vi "CSM with allowed message list.vi"(7 "Name (\"\" to Use Uuid)":string="Event CSM Tiny") -> ()   [LabVIEW 2017]
doc: "------------- lvcsm -------------\n[CSMStates]\nItem 0 = \"Event Structure\"\nItem 1 = \"Idle\"\nItem 2 = \"CSM Documentation\"\nItem 3 = \"VI Reference\"\nItem 4 = \"Error Handler\"\nItem 5 = \"Critical Error\"\nItem 6 = \"Target Busy Error\"\nItem 7 = \"Target Error\"\nItem 8 = \"Target Timeout Error\"\nItem 9 = \"Async Response\"\nItem 10 = \"Response\"\nItem 11 = \"Async Message Posted\"\nItem 12 = \"Initialize Core Data\"\nItem 13 = \"Exit\"\nItem 14 = \"Data: Initialize\"\nItem 15 = \"Data: Cleanup\"\nItem 16 = \"Events: Register\"\nItem 17 = \"Events: Unregister\"\nItem 18 = \"UI: Initialize\"\nItem 19 = \"UI: Cursor Set\"\nItem 20 = \"UI: Front Panel State\"\nItem 21 = \"Macro: Initialize\"\nItem 22 = \"Macro: Exit\"\nItem 23 = \"API: API1\"\nItem 24 = \"API: API2\"\nItem 25 = \"DoSth: DoA\"\nItem 26 = \"DoSth: DoB\"\n\n[CSMStatus]\nItem 0 = \"Error Occurred@Error Handler\""
uses:
  user.lib/_NEVSTOP/Communicable State Machine(CSM)/AdvanceAPI/CSM - Revert Arguments-Safe String.vi
  user.lib/_NEVSTOP/Communicable State Machine(CSM)/AdvanceAPI/CSM - Break Down Multiple States String.vi
  user.lib/_NEVSTOP/Communicable State Machine(CSM)/AdvanceAPI/CSM - Compact Multiple States.vi
  user.lib/_NEVSTOP/Communicable State Machine(CSM)/AdvanceAPI/CSM - Make String Arguments Safe.vi
  user.lib/_NEVSTOP/Communicable State Machine(CSM)/AdvanceAPI/CSM - Keywords.vi
  user.lib/_NEVSTOP/Communicable State Machine(CSM)/_Shared/Trim Single-line Text.vi
  user.lib/_NEVSTOP/Communicable State Machine(CSM)/Communicable State Machine.lvlib
panel:
  in  "Init State(\"Macro: Initialize\")":string="Macro: Initialize"
  out "State History":string
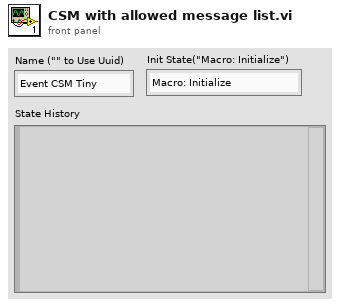
[diagram p1: front panel]
types:
  T1 = enum32{"Invalid", "Standard", "Closed", "Hidden", "Minimized", "Maximized"}
  T2 = enum32{"invalid app kind", "Development System", "Run Time System", "Student Edition", "Embedded LabVIEW", "Evaluation", "Custom"}
  T3 = typedef "Communicable State Machine.lvlib/_CSM_Response Source Message.ctl" = cluster{"‘State":string, "’Arguments":string, "’Error":errorcluster}
  T4 = cluster{"Current VI Reference":refnum<vi>, "Close Panel on Exit?":bool}
  T5 = cluster{"Core":cluster{"Current VI Reference":refnum<vi>, "Close Panel on Exit?":bool}, "Your Boolean data":bool, "Your string data":string}
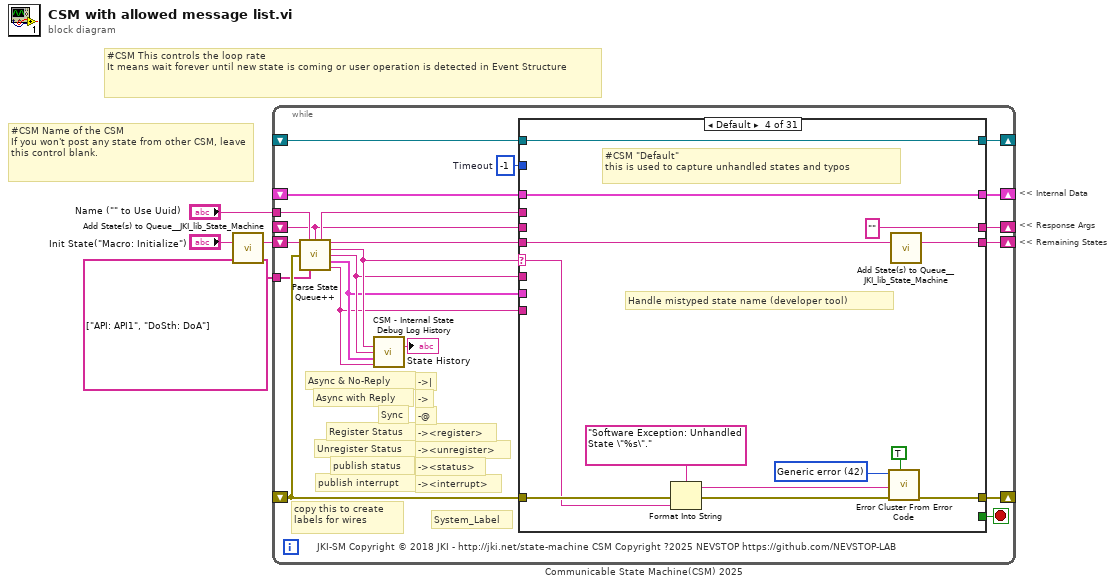
[diagram p0: block diagram]
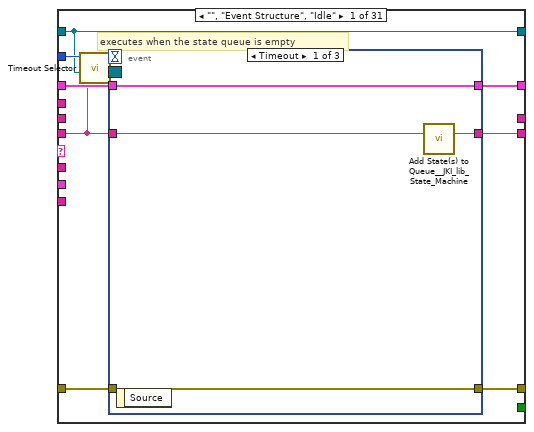
[diagram p2: hidden frame]
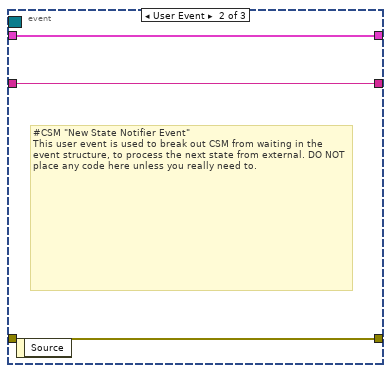
[diagram p3: hidden frame]
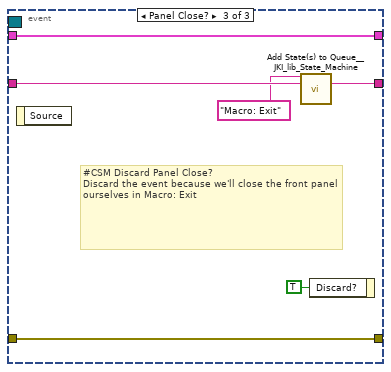
[diagram p4: hidden frame]
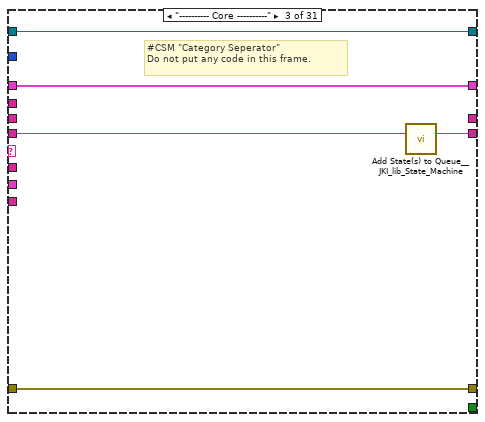
[diagram p6: hidden frame]
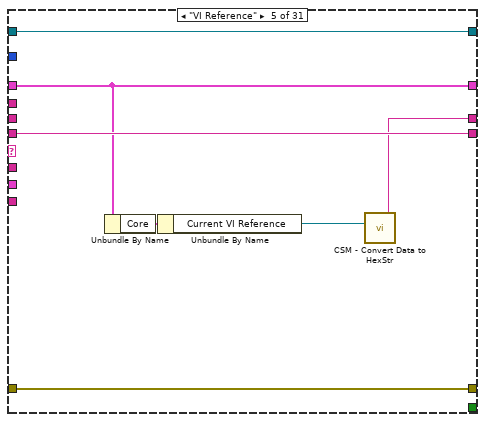
[diagram p7: hidden frame]
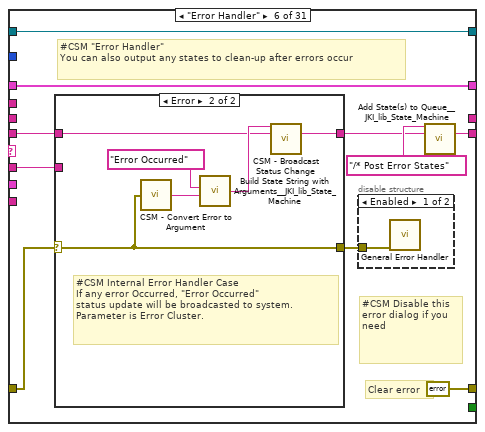
[diagram p8: hidden frame]
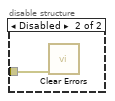
[diagram p9: hidden frame]
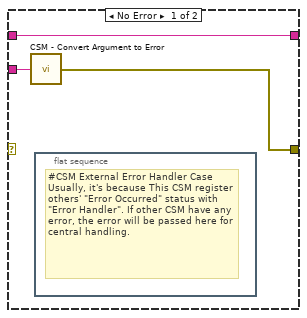
[diagram p10: hidden frame]
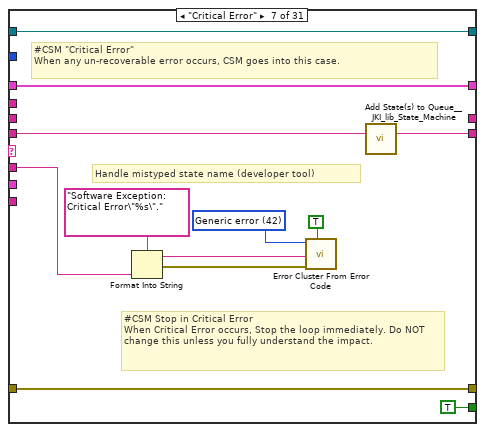
[diagram p11: hidden frame]
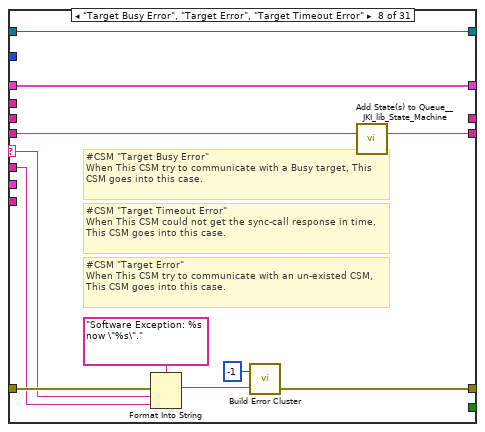
[diagram p12: hidden frame]
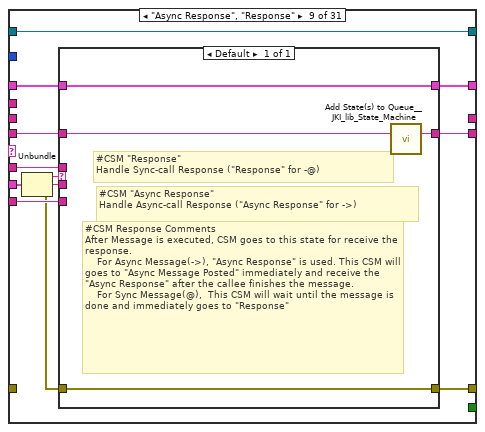
[diagram p13: hidden frame]
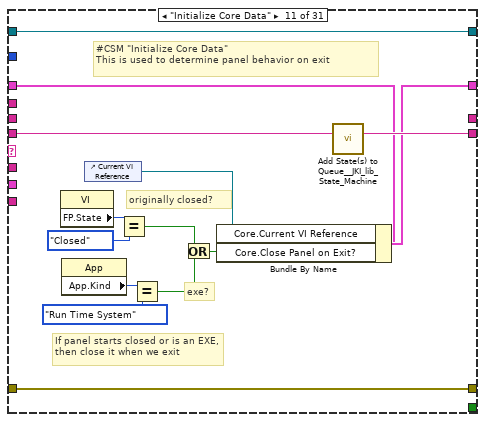
[diagram p15: hidden frame]
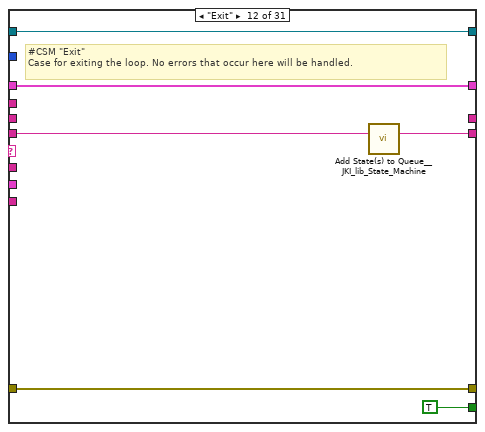
[diagram p16: hidden frame]
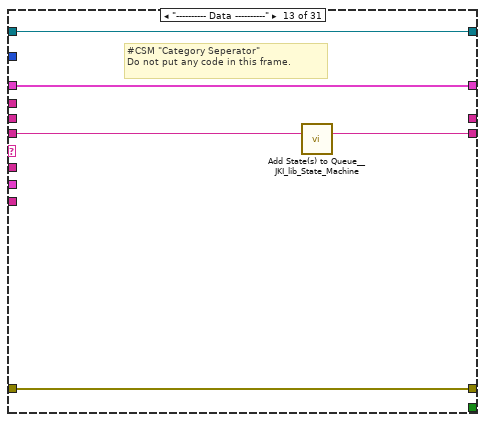
[diagram p17: hidden frame]
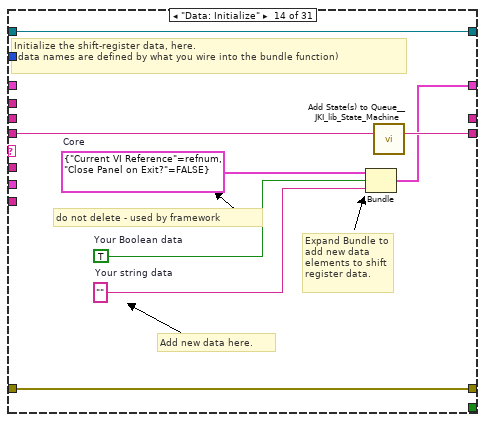
[diagram p18: hidden frame]
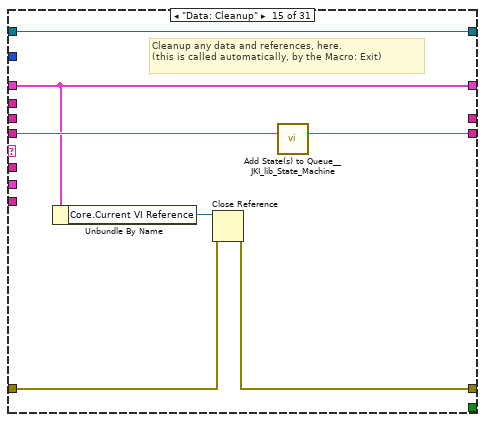
[diagram p19: hidden frame]
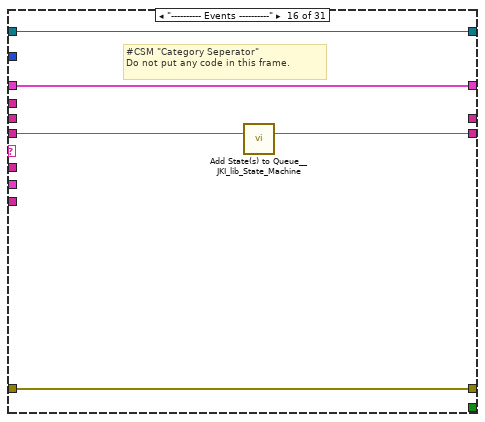
[diagram p20: hidden frame]
diagram:
  # "#CSM Name of the CSM\nIf you won't post any state from other CSM, leave this control blank."
  # "#CSM This controls the loop rate\nIt means wait forever until new state is coming or user operation is detected in Event Structure"
  # "<< Internal Data"
  # "<< Response Args"
  # "<< Remaining States"
  n1 = call <vilib>:"Add State(s) to Queue__JKI_lib_State_Machine.vi"("State(s) in (\"\")"="Init State(\"Macro: Initialize\")") -> ("States Out"=w4:string)  [unwired: 14 in]
  n2 = while "Communicable State Machine(CSM) 2025" {
    shift-right: [w20] -> _
    shift-left: _ -> [w19]
    shift-right: [w23] -> _
    shift-left: _ -> [w17]
    shift-right: [w22] -> _
    shift-left: w4 -> [w24]
    tunnel: "Name (\"\" to Use Uuid)" -> [w13]
    shift-right: [w16] -> _
    shift-left: _ -> [w7]
    shift-right: [w15] -> _
    shift-left: _ -> [w14]
    tunnel: string[] ["API: API1", "DoSth: DoA"] ("Allowed Messages(Empty for all)") -> [w6]
    stop <- w21 stop-if-true
    w18 = -1  # Timeout
    # "-><interrupt>"
    # "-><status>"
    # "-><unregister>"
    # "-><register>"
    # "-@"
    # "->"
    # "->|"
    # "publish interrupt"
    # "publish status"
    # "Unregister Status"
    # "Register Status"
    # "Sync"
    # "Async with Reply"
    # "Async & No-Reply"
    # "copy this to create labels for wires"
    # "System_Label"
    # "JKI-SM Copyright © 2018 JKI - http://jki.net/state-machine CSM Copyright ?2025 NEVSTOP https://github.com/NEVSTOP-LAB"
    n3 = call "Parse State Queue++.vi"("State Queue"=w24, "Name (\"\" to Use UUID)"=w13, "Response Arguments"=w7, "Previous Error"=w17, "Allowed Messages (Empty for All)"=w6) -> ("Name Used"=w8:string, "Remaining States"=w25:string, "Current State"=w12:string, "Arguments"=w11:string, ">> Response Source Message >>"=w10:T3, ">> Source CSM >>"=w9:string)  [unwired: 5 in]
    n4 = call "CSM - Internal State Debug Log History.vi"("State"=w12, "Arguments (\"\")"=w11, ">> Response Source Message >>"=w10, "Source (\"\")"=w9) -> ("Debug Log"=→"State History":string)  [unwired: 11 in]
    n5 = case shown="Default" w12 {
      selector: w12 -> [_ _ _ w59 _ _ _ w113 _ _ _ _ _ _ _ _ _ _ _ _ _ _ _ _ _ _ _ _ _ _ _]
      tunnel: w25 -> [w26 w50 w56 w63 w75 w81 w107 w115 w126 w139 w154 w160 w165 w173 w180 w185 w192 w196 w202 w207 w214 w230 w300 w306 w317 w320 w325 w331 w339 w345 w351]
      tunnel: w11 -> [_ _ _ _ _ w80 w100 w114 w125 _ _ _ _ _ _ _ _ _ _ _ w209 w224 _ _ _ _ _ w328 _ _ _]
      tunnel: w19 -> [w33 w49 w53 w61 w74 w85 w108 w117 w128 w138 w147 w158 w162 _ w175 w182 w191 w195 w199 w205 w212 w226 w297 w303 w314 w319 w324 w330 w336 w342 w348]
      tunnel: [w32 w51 w54 w65 w76 errorcluster {"status"=FALSE, "code"=0, "source"=""} ("error out") w109 w111 w131 w140 w151 w157 w163 w170 w176 w183 w186 w194 w200 w204 w210 w227 w298 w304 w315 w321 w326 w332 w337 w343 w349] -> w23
      tunnel: w17 -> [w31 w51 w54 w64 w76 w82 w109 w119 _ w140 w151 w157 w163 w170 w177 w183 _ w197 w200 w204 w211 w228 w298 w304 w315 w321 w326 w332 w337 w343 w349]
      tunnel: [w34 w50 w55 w62 w75 w77 w106 w118 w127 w139 w153 w159 w164 w172 w179 w184 w192 w196 w201 w206 w213 w229 w299 w305 w316 w320 w325 w331 w338 w344 w350] -> w22
      tunnel: [_ _ _ _ _ _ TRUE _ _ _ _ TRUE _ _ _ _ _ _ _ _ _ _ _ _ _ _ _ _ _ _ _] -> w21
      tunnel: [w30 w49 w53 w61 w74 w85 w108 w117 w129 w138 w152 w158 w162 w171 w175 w182 w191 w195 w199 w205 w212 w226 w297 w303 w314 w319 w324 w330 w336 w342 w348] -> w20
      tunnel: w18 -> [w29 _ _ _ _ _ _ _ _ _ _ _ _ _ _ _ _ _ _ _ _ _ _ _ _ _ _ _ _ _ _]
      tunnel: w9 -> [_ _ _ _ _ _ _ _ w123 _ _ _ _ _ _ _ _ _ _ _ _ _ _ _ _ _ _ _ _ _ _]
      tunnel: w10 -> [_ _ _ _ _ _ _ _ w130 _ _ _ _ _ _ _ _ _ _ _ _ _ _ _ _ _ _ _ _ _ _]
      tunnel: [_ _ _ "" w70 _ _ _ _ _ _ _ _ _ _ _ _ _ _ _ _ _ _ _ _ _ "API1 Response" w327 _ "DoA Finished" "DoB Finished"] -> w16
      tunnel: [w28 w48 w52 w57 w73 w84 w98 w116 w132 w137 w141 w155 w161 w166 w174 w181 w190 w193 w198 w203 w208 w223 w296 w301 w307 w318 w323 w329 w335 w341 w347] -> w15
      tunnel: w14 -> [w28 w48 w52 w57 w73 w84 w98 w116 w132 w137 w141 w155 w161 w166 w174 w181 _ w193 w198 w203 w208 w223 w296 w301 w307 w318 w323 w329 w335 w341 w347]
      tunnel: w8 -> [_ _ _ _ _ _ _ _ _ _ _ _ _ _ _ _ w189 _ _ _ _ _ _ _ _ _ _ _ _ _ _]
      tunnel: w7 -> [_ _ _ _ _ _ _ _ _ _ _ _ _ _ _ _ _ _ _ _ _ _ _ _ _ _ _ _ _ _ _]
      frame "", "Event Structure", "Idle" {
        # "executes when the state queue is empty"
        n6 = call "Timeout Selector.vi"("Remaining States"=w26, "Timeout Expected"=w29) -> ("Timeout"=w27:i32)  [unwired: 5 in]
        n7 = event shown="[0] Timeout" {
          selector: w28 -> [_ _ _]
          dyn-events: _ -> [_ _ _]
          timeout: w27 -> [_ _ _]
          tunnel: w26 -> [w38 w40 w47]
          tunnel: [w37 w40 w46] -> w34
          tunnel: w33 -> [w35 w41 w44]
          tunnel: [w36 w39 w45] -> w32
          tunnel: w31 -> [w36 w39 w45]
          tunnel: [w35 w41 w44] -> w30
          event Timeout {
            n8 = event-data() -> ()  [unwired: 1 in, 1 out]
            n9 = call <vilib>:"Add State(s) to Queue__JKI_lib_State_Machine.vi"("State(s) in (\"\")"=w38) -> ("States Out"=w37:string)  [unwired: 14 in]
          }
          event User Event {
            # "#CSM \"New State Notifier Event\"\nThis user event is used to break out CSM from waiting in the event structure, to process the next state from external. DO NOT place any code here unless you really need to."
            n10 = event-data() -> ()  [unwired: 1 in, 1 out]
          }
          event Panel Close? {
            # "#CSM Discard Panel Close?\nDiscard the event because we'll close the front panel ourselves in Macro: Exit"
            n11 = event-data() -> ()  [unwired: 1 in, 1 out]
            n12 = call <vilib>:"Add State(s) to Queue__JKI_lib_State_Machine.vi"("State(s) in Front (\"\")"="Macro: Exit", "State(s) in (\"\")"=w47) -> ("States Out"=w46:string)  [unwired: 13 in]
            n13 = event-data("Discard?"=TRUE) -> ()  [unwired: 1 in, 1 out]
          }
        }
      }
      frame "CSM Documentation" {
        # "#CSM README FIRST\n\nCSM is a LabVIEW application framework that builds upon JKI State Machine (JKISM). It follows the pattern of JKISM and extends the keywords to describe message communication between CSM modules, including concepts such as Sync-Message, Async-Message, Subscription/Unsubscription of status - essential elements for creating reusable code modules. For more information, please visit the CSM wiki: https://github.com/NEVSTOP-LAB/JKI-State-Machine-Plus-Plus/wiki\n\nFor instructions on JKI State Machine, visit: http://jki.net/state-machine/\nFor information about CSM, visit: https://github.com/NEVSTOP-LAB"
        # "#CSM \"Documentation\"\nCase for holding CSM Documenation"
      }
      frame "---------- Core ----------" {
        # "#CSM \"Category Seperator\"\nDo not put any code in this frame."
        n14 = call <vilib>:"Add State(s) to Queue__JKI_lib_State_Machine.vi"("State(s) in (\"\")"=w56) -> ("States Out"=w55:string)  [unwired: 14 in]
      }
      frame Default {
        w68 = 42 items=["No error", "Argument error", "Memory is full", "Out of zone", "End of file", "File already open", "Generic file I/O error", "File not found", "File permission error", "Disk is full", "Duplicate path", "Too many files open", "System feature not enabled", "Resource file not found", "Cannot add resource", "Resource not found", "Image not found", "Image memory error", "Pen does not exist", "Config type invalid", "Config token not found", "Config parse error", "Config memory error", "Bad external code format", "Bad external code offset", "External code not present", "Null window", "Destroy window error", "Null menu", "Print aborted", "Bad print record", "Print driver error", "Windows error during printing", "Memory error during printing", "Print dialog error", "Generic print error", "Invalid device refnum", "Device not found", "Device parameter error", "Device unit error", "Cannot open device", "Device call aborted", "Generic error", "Cancelled by user", "Object ID too low", "Object ID too high", "Object not in heap", "Unknown heap", "Unknown object (invalid DefProc)", "Unknown object (DefProc not in table)", "Message out of range", "Invalid (null) method", "Unknown message", "Manager call not supported", "Bad address", "Network operation in progress", "Network operation timed out", "Connection is busy", "Network attribute not supported", "Network error", "Address in use", "System out of memory", "Connection aborted", "Connection refused", "Not connected", "Already connected", "Connection closed", "Initialization error (interapplication manager)", "Bad occurrence", "Wait on unbound occurrence handler", "Occurrence queue overflow", "Datalog type conflict", "Unused", "Unrecognized type (interapplication manager)", "Memory corrupt", "Failed to make temporary DLL", "Old CIN version", "Drag socket not found", "Failed to load drop-object", "Failed to register OLE object", "Failed to release OLE object", "Format specifier type mismatch", "Unknown format specifier", "Too few format specifiers", "Too many format specifiers", "Scan failed", "Newer CIN version", "Error converting to variant", "Runtime menu error", "Password tampered", "Variant attribute not found", "Incompatible variant data type", "Event data is not available", "Event Store is not present", "Occurrence is not found", "Event Queue is not created", "Event info is not available", "Refnum passed is NULL", "Error retrieving Class GUID", "Error retrieving CoClass GUID", "Error retrieving TypeLib GUID.", "Bad built application magic bytes.", "Specific driver is different from the specific driver associated with the Logical Name.", "There is no session opened to the class driver.", "Max Error", "MAX - Error with config objects", "MAX - Error loading configuration", "MAX - Group not supported"]
        # "#CSM \"Default\"\nthis is used to capture unhandled states and typos"
        # "Handle mistyped state name (developer tool)"
        n15 = Format Into String(format string="Software Exception: Unhandled State \"%s\"." ("message"), error in=w64, w59) -> (resulting string=w67:string, error out=w66:errorcluster)  [unwired: 1 in]
        n16 = call <vilib>:"Error Cluster From Error Code.vi"("show call chain? (False)"=TRUE, "error in (no error)"=w66, "error message (\"\")"=w67, "error code (0)"=w68) -> ("error out"=w65:errorcluster)  [unwired: 5 in]
        n17 = call <vilib>:"Add State(s) to Queue__JKI_lib_State_Machine.vi"("State(s) in (\"\")"=w63) -> ("States Out"=w62:string)  [unwired: 14 in]
      }
      frame "VI Reference" {
        n18 = Unbundle By Name(w74) -> ("Core"=w72:T4)
        n19 = Unbundle By Name(w72) -> ("Current VI Reference"=w71:refnum<vi>)
        n20 = call "CSM - Convert Data to HexStr.vi"("Variant"=w71) -> ("HEX String (0-9,A-F)"=w70:string)  [unwired: 8 in]
      }
      frame "Error Handler" {
        # "#CSM Disable this error dialog if you need"
        # "#CSM \"Error Handler\"\nYou can also output any states to clean-up after errors occur"
        # "Clear error"
        n21 = case shown="Error" w82 {
          selector: w82 -> [_ w92]
          tunnel: [w91 w94] -> w78
          tunnel: w81 -> [w91 w93]
          tunnel: w80 -> [w90 _]
          tunnel: [w89 w92] -> w83
          frame No Error {
            n22 = call "CSM - Convert Argument to Error.vi"("Argument"=w90) -> ("Error"=w89:errorcluster)  [unwired: 4 in]
            n23 = flat-sequence {
              frame #0 {
                # "#CSM External Error Handler Case\nUsually, it's because This CSM register others' \"Error Occurred\" status with \"Error Handler\". If other CSM have any error, the error will be passed here for central handling."
              }
            }
          }
          frame Error {
            # "#CSM Internal Error Handler Case \nIf any error Occurred, \"Error Occurred\" \nstatus update will be broadcasted to system.\nParameter is Error Cluster."
            n24 = call "CSM - Convert Error to Argument.vi"("Error"=w92) -> ("Argument"=w96:string)  [unwired: 4 in]
            n25 = call <vilib>:"Build State String with Arguments__JKI_lib_State_Machine.vi"("Arguments (\"\")"=w96, "State"="Error Occurred" ("Status with Arguments")) -> ("State with Arguments"=w95:string)  [unwired: 4 in]
            n26 = call "CSM - Broadcast Status Change.vi"("Status With Arguments"=w95, "State Queue"=w93) -> ("Remaining States"=w94:string)  [unwired: 13 in]
          }
        }
        n27 = disable-structure shown="Enabled" {
          disable-tunnel: w83 -> [w87 w88]
          frame Enabled {
            n28 = call <vilib>:"General Error Handler.vi"("error in (no error)"=w87) -> ()  [unwired: 10 in, 5 out]
          }
          frame Disabled {
            n29 = call <vilib>:"Clear Errors.vi"("error in (no error)"=w88) -> ()  [unwired: 5 in, 2 out]
          }
        }
        n30 = call <vilib>:"Add State(s) to Queue__JKI_lib_State_Machine.vi"("State(s) in Front (\"\")"="/* Post Error States", "State(s) in (\"\")"=w78) -> ("States Out"=w77:string)  [unwired: 13 in]
      }
      frame "Critical Error" {
        w104 = 42 items=["No error", "Argument error", "Memory is full", "Out of zone", "End of file", "File already open", "Generic file I/O error", "File not found", "File permission error", "Disk is full", "Duplicate path", "Too many files open", "System feature not enabled", "Resource file not found", "Cannot add resource", "Resource not found", "Image not found", "Image memory error", "Pen does not exist", "Config type invalid", "Config token not found", "Config parse error", "Config memory error", "Bad external code format", "Bad external code offset", "External code not present", "Null window", "Destroy window error", "Null menu", "Print aborted", "Bad print record", "Print driver error", "Windows error during printing", "Memory error during printing", "Print dialog error", "Generic print error", "Invalid device refnum", "Device not found", "Device parameter error", "Device unit error", "Cannot open device", "Device call aborted", "Generic error", "Cancelled by user", "Object ID too low", "Object ID too high", "Object not in heap", "Unknown heap", "Unknown object (invalid DefProc)", "Unknown object (DefProc not in table)", "Message out of range", "Invalid (null) method", "Unknown message", "Manager call not supported", "Bad address", "Network operation in progress", "Network operation timed out", "Connection is busy", "Network attribute not supported", "Network error", "Address in use", "System out of memory", "Connection aborted", "Connection refused", "Not connected", "Already connected", "Connection closed", "Initialization error (interapplication manager)", "Bad occurrence", "Wait on unbound occurrence handler", "Occurrence queue overflow", "Datalog type conflict", "Unused", "Unrecognized type (interapplication manager)", "Memory corrupt", "Failed to make temporary DLL", "Old CIN version", "Drag socket not found", "Failed to load drop-object", "Failed to register OLE object", "Failed to release OLE object", "Format specifier type mismatch", "Unknown format specifier", "Too few format specifiers", "Too many format specifiers", "Scan failed", "Newer CIN version", "Error converting to variant", "Runtime menu error", "Password tampered", "Variant attribute not found", "Incompatible variant data type", "Event data is not available", "Event Store is not present", "Occurrence is not found", "Event Queue is not created", "Event info is not available", "Refnum passed is NULL", "Error retrieving Class GUID", "Error retrieving CoClass GUID", "Error retrieving TypeLib GUID.", "Bad built application magic bytes.", "Specific driver is different from the specific driver associated with the Logical Name.", "There is no session opened to the class driver.", "Max Error", "MAX - Error with config objects", "MAX - Error loading configuration", "MAX - Group not supported"]
        # "#CSM Stop in Critical Error\nWhen Critical Error occurs, Stop the loop immediately. Do NOT change this unless you fully understand the impact."
        # "#CSM \"Critical Error\"\nWhen any un-recoverable error occurs, CSM goes into this case."
        # "Handle mistyped state name (developer tool)"
        n31 = Format Into String(format string="Software Exception: Critical Error\"%s\"." ("message"), w100) -> (resulting string=w103:string, error out=w102:errorcluster)  [unwired: 2 in]
        n32 = call <vilib>:"Error Cluster From Error Code.vi"("show call chain? (False)"=TRUE, "error in (no error)"=w102, "error message (\"\")"=w103, "error code (0)"=w104) -> ()  [unwired: 5 in, 1 out]
        n33 = call <vilib>:"Add State(s) to Queue__JKI_lib_State_Machine.vi"("State(s) in (\"\")"=w107) -> ("States Out"=w106:string)  [unwired: 14 in]
      }
      frame "Target Busy Error", "Target Error", "Target Timeout Error" {
        # "#CSM \"Target Error\"\nWhen This CSM try to communicate with an un-existed CSM, This CSM goes into this case."
        # "#CSM \"Target Timeout Error\"\nWhen This CSM could not get the sync-call response in time, This CSM goes into this case."
        # "#CSM \"Target Busy Error\"\nWhen This CSM try to communicate with a Busy target, This CSM goes into this case."
        n34 = Format Into String(format string="Software Exception: %s now \"%s\"." ("message"), error in=w119, w113, w114) -> (resulting string=w112:string)  [unwired: 1 in, 1 out]
        n35 = call "Build Error Cluster.vi"("String to Prepend to Source (\"\")"=w112, "Code"=-1 ("code")) -> ("error out"=w111:errorcluster)
        n36 = call <vilib>:"Add State(s) to Queue__JKI_lib_State_Machine.vi"("State(s) in (\"\")"=w115) -> ("States Out"=w118:string)  [unwired: 14 in]
      }
      frame "Async Response", "Response" {
        n37 = Unbundle(w130) -> ("‘State"=w124:string, "’Arguments"=w122:string, "’Error"=w121:errorcluster)
        n38 = case shown="Default" w124 {
          tunnel: [w136] -> w131
          tunnel: w121 -> [w136]
          tunnel: [w135] -> w129
          tunnel: w128 -> [w135]
          tunnel: [w133] -> w127
          tunnel: w126 -> [w134]
          tunnel: w125 -> [_]
          tunnel: w123 -> [_]
          tunnel: w122 -> [_]
          frame Default {
            # "#CSM Response Comments\nAfter Message is executed, CSM goes to this state for receive the response.\n    For Async Message(->), \"Async Response\" is used. This CSM will goes to \"Async Message Posted\" immediately and receive the \"Async Response\" after the callee finishes the message.\n    For Sync Message(@),  This CSM will wait until the message is done and immediately goes to \"Response\""
            # "#CSM \"Async Response\"\nHandle Async-call Response (\"Async Response\" for ->)"
            # "#CSM \"Response\"\nHandle Sync-call Response (\"Response\" for -@)"
            n39 = call <vilib>:"Add State(s) to Queue__JKI_lib_State_Machine.vi"("State(s) in (\"\")"=w134) -> ("States Out"=w133:string)  [unwired: 14 in]
          }
        }
      }
      frame "Async Message Posted" {
        # "#CSM \"Async Message Posted\"\nAfter Async Message is posted (-> or ->| ), CSM goes to this state for post-action.\nYou can use Argument - State to tell which Async Message is called."
      }
      frame "Initialize Core Data" {
        # "#CSM \"Initialize Core Data\"\nThis is used to determine panel behavior on exit"
        # "originally closed?"
        # "exe?"
        # "If panel starts closed or is an EXE, then close it when we exit"
        n40 = property class="VI"() -> ("FP.State"=w144:T1)  [unwired: 2 in, 2 out]
        n41 = property class="App"() -> ("App.Kind"=w150:T2)  [unwired: 2 in, 2 out]
        n42 = control-ref of="Current VI Reference"() -> (w145:refnum<vi>)
        n43 = Equal?(x=w144, y=T1."Closed" ("Front Panel Window:State")) -> (x = y?=w142:bool)
        n44 = Equal?(x=w150, y=T2."Run Time System" ("Application:Kind")) -> (x = y?=w148:bool)
        n45 = Or(x=w142, y=w148) -> (x .or. y?=w146:bool)
        n46 = Bundle By Name(cluster=w147, "Core.Current VI Reference"=w145, "Core.Close Panel on Exit?"=w146) -> (w152:T5)
        n47 = call <vilib>:"Add State(s) to Queue__JKI_lib_State_Machine.vi"("State(s) in (\"\")"=w154) -> ("States Out"=w153:string)  [unwired: 14 in]
      }
      frame "Exit" {
        # "#CSM \"Exit\"\nCase for exiting the loop. No errors that occur here will be handled."
        n48 = call <vilib>:"Add State(s) to Queue__JKI_lib_State_Machine.vi"("State(s) in (\"\")"=w160) -> ("States Out"=w159:string)  [unwired: 14 in]
      }
      frame "---------- Data ----------" {
        # "#CSM \"Category Seperator\"\nDo not put any code in this frame."
        n49 = call <vilib>:"Add State(s) to Queue__JKI_lib_State_Machine.vi"("State(s) in (\"\")"=w165) -> ("States Out"=w164:string)  [unwired: 14 in]
      }
      frame "Data: Initialize" {
        w167 = T4 {"Current VI Reference"=refnum, "Close Panel on Exit?"=FALSE}  # Core
        w169 = TRUE  # Your Boolean data
        w168 = ""  # Your string data
        # "do not delete - used by framework"
        # "Expand Bundle to add new data elements to shift register data."
        # "Add new data here."
        # "Initialize the shift-register data, here.\n(data names are defined by what you wire into the bundle function)"
        n50 = Bundle("Core"=w167, "Your Boolean data"=w169, "Your string data"=w168) -> (w171:T5)  [unwired: 1 in]
        n51 = call <vilib>:"Add State(s) to Queue__JKI_lib_State_Machine.vi"("State(s) in (\"\")"=w173) -> ("States Out"=w172:string)  [unwired: 14 in]
      }
      frame "Data: Cleanup" {
        # "Cleanup any data and references, here.\n(this is called automatically, by the Macro: Exit)"
        n52 = Unbundle By Name(w175) -> ("Core.Current VI Reference"=w178:refnum<vi>)
        n53 = Close Reference(reference=w178, error in (no error)=w177) -> (error out=w176:errorcluster)
        n54 = call <vilib>:"Add State(s) to Queue__JKI_lib_State_Machine.vi"("State(s) in (\"\")"=w180) -> ("States Out"=w179:string)  [unwired: 14 in]
      }
      frame "---------- Events ----------" {
        # "#CSM \"Category Seperator\"\nDo not put any code in this frame."
        n55 = call <vilib>:"Add State(s) to Queue__JKI_lib_State_Machine.vi"("State(s) in (\"\")"=w185) -> ("States Out"=w184:string)  [unwired: 14 in]
      }
      frame "Events: Register" {
        # "#CSM \"Events: Register\"\nRegister user event. New Message Event is registered to break CSM waiting in event structure by default."
        # "#CSM Register New Message Event\nRegister message event to break Waiting in Event structure."
        n56 = call "CSM - Get New State Notifier Event.vi"("Name (\"\" to Use UUID) In"=w189) -> ("error out"=w187:errorcluster, "New State Notifier Event"=w188:refnum<user-event>)  [unwired: 9 in]
        n57 = register-events(error in=w187, w188) -> (reference out=w190:refnum<event-registration>, error out=w186:errorcluster)  [unwired: 1 in]
      }
      frame "Events: Unregister" {
        # "#CSM \"Events: Unregister\"\nUnregister user event."
        n58 = Unregister For Events(event registration refnum=w193, error in=w197) -> (error out=w194:errorcluster)
      }
      frame "---------- UI ----------" {
        # "#CSM \"Category Seperator\"\nDo not put any code in this frame."
        n59 = call <vilib>:"Add State(s) to Queue__JKI_lib_State_Machine.vi"("State(s) in (\"\")"=w202) -> ("States Out"=w201:string)  [unwired: 14 in]
      }
      frame "UI: Initialize" {
        # "#CSM \"UI: Initialize\"\nInitialize the User Interface, here.\n(this is called automatically, by the Macro: Init)"
        n60 = call <vilib>:"Add State(s) to Queue__JKI_lib_State_Machine.vi"("State(s) in (\"\")"=w207) -> ("States Out"=w206:string)  [unwired: 14 in]
      }
      frame "UI: Cursor Set" {
        # "#CSM \"UI: Cursor Set\"\nSet and Unset Cursor Busy.\n(Usage: \"UI: Cursor Set >> Busy|Idle\")"
        # "Argument"
        n61 = disable-structure shown="TARGET_TYPE!=Windows" {
          disable-tunnel: w211 -> [w217 w222]
          disable-tunnel: [w216 w222] -> w210
          disable-tunnel: w209 -> [w215 _]
          frame condition #0 (active) {
            n62 = case shown="\"Idle\", Default" w215 {
              tunnel: w217 -> [w219 w221]
              tunnel: [w218 w220] -> w216
              frame "Idle", Default {
                n63 = call <vilib>:"Unset Busy.vi"("error in (no error)"=w219) -> ("error out"=w218:errorcluster)  [unwired: 10 in]
              }
              frame "Busy" {
                n64 = call <vilib>:"Set Busy.vi"("error in (no error)"=w221) -> ("error out"=w220:errorcluster)  [unwired: 9 in, 1 out]
              }
            }
          }
          frame condition #1 {
          }
        }
        n65 = call <vilib>:"Add State(s) to Queue__JKI_lib_State_Machine.vi"("State(s) in (\"\")"=w214) -> ("States Out"=w213:string)  [unwired: 14 in]
      }
      frame "UI: Front Panel State" {
        # "#CSM \"UI: Front Panel State\"\nSet Front Panel Open or Closed\n(Usage: \"UI: Front Panel State >> Open|Close\")"
        # "Argument"
        n66 = Unbundle By Name(w226) -> ("Core.Current VI Reference"=w225:refnum<vi>)
        n67 = call <vilib>:"Add State(s) to Queue__JKI_lib_State_Machine.vi"("State(s) in (\"\")"=w230) -> ("States Out"=w229:string)  [unwired: 14 in]
        n68 = case shown="\"Close\", \"Closed\"" w224 {
          tunnel: w228 -> [w236 w251 w262 w275 w288]
          tunnel: [w238 w252 w264 w277 w290] -> w227
          tunnel: w225 -> [w237 w249 w263 w276 w289]
          frame "Open", "Standard", Default {
            w231 = T1."Standard" ("State")
            n69 = property class="VI"(reference=w237, error in=w236) -> (reference out=w234:refnum<vi>, error out=w235:errorcluster, "FP.State"=w233:T1)
            n70 = Not Equal?(x=w233, y=w231) -> (x != y?=w232:bool)
            n71 = case shown="True" w232 {
              tunnel: [w242 w244] -> w238
              tunnel: w235 -> [w241 w244]
              tunnel: w234 -> [w240 _]
              tunnel: w231 -> [w239 _]
              frame True {
                n72 = invoke class="VI" method="FP.Open"(reference=w240, error in=w241, "Activate"=TRUE, "State"=w239) -> (error out=w242:errorcluster)  [unwired: 1 in, 4 out]
              }
              frame False {
              }
            }
          }
          frame "Close", "Closed" {
            n73 = property class="VI"(reference=w249, error in=w251) -> (reference out=w248:refnum<vi>, error out=w250:errorcluster, "FP.State"=w246:T1)
            n74 = Not Equal?(x=w246, y=T1."Closed" ("Front Panel Window:State")) -> (x != y?=w245:bool)
            n75 = case shown="False" w245 {
              tunnel: [w253 w256] -> w252
              tunnel: w250 -> [w253 w255]
              tunnel: w248 -> [_ w254]
              frame False {
              }
              frame True {
                n76 = invoke class="VI" method="FP.Close"(reference=w254, error in=w255) -> (error out=w256:errorcluster)  [unwired: 1 in, 2 out]
              }
            }
          }
          frame "Hidden", "Hide" {
            w257 = T1."Hidden" ("State")
            n77 = property class="VI"(reference=w263, error in=w262) -> (reference out=w260:refnum<vi>, error out=w261:errorcluster, "FP.State"=w259:T1)
            n78 = Not Equal?(x=w259, y=w257) -> (x != y?=w258:bool)
            n79 = case shown="True" w258 {
              tunnel: [w268 w269] -> w264
              tunnel: w261 -> [w267 w269]
              tunnel: w260 -> [w266 _]
              tunnel: w257 -> [w265 _]
              frame True {
                n80 = invoke class="VI" method="FP.Open"(reference=w266, error in=w267, "State"=w265) -> (error out=w268:errorcluster)  [unwired: 2 in, 4 out]
              }
              frame False {
              }
            }
          }
          frame "Minimize", "Minimized" {
            w270 = T1."Minimized" ("State")
            n81 = property class="VI"(reference=w276, error in=w275) -> (reference out=w273:refnum<vi>, error out=w274:errorcluster, "FP.State"=w272:T1)
            n82 = Not Equal?(x=w272, y=w270) -> (x != y?=w271:bool)
            n83 = case shown="True" w271 {
              tunnel: [w281 w282] -> w277
              tunnel: w274 -> [w280 w282]
              tunnel: w273 -> [w279 _]
              tunnel: w270 -> [w278 _]
              frame True {
                n84 = invoke class="VI" method="FP.Open"(reference=w279, error in=w280, "State"=w278) -> (error out=w281:errorcluster)  [unwired: 2 in, 4 out]
              }
              frame False {
              }
            }
          }
          frame "Maximize", "Maximized" {
            w283 = T1."Maximized" ("State")
            n85 = property class="VI"(reference=w289, error in=w288) -> (reference out=w286:refnum<vi>, error out=w287:errorcluster, "FP.State"=w285:T1)
            n86 = Not Equal?(x=w285, y=w283) -> (x != y?=w284:bool)
            n87 = case shown="True" w284 {
              tunnel: [w294 w295] -> w290
              tunnel: w287 -> [w293 w295]
              tunnel: w286 -> [w292 _]
              tunnel: w283 -> [w291 _]
              frame True {
                n88 = invoke class="VI" method="FP.Open"(reference=w292, error in=w293, "State"=w291) -> (error out=w294:errorcluster)  [unwired: 2 in, 4 out]
              }
              frame False {
              }
            }
          }
        }
      }
      frame "---------- Macro ----------" {
        # "#CSM \"Category Seperator\"\nDo not put any code in this frame."
        n89 = call <vilib>:"Add State(s) to Queue__JKI_lib_State_Machine.vi"("State(s) in (\"\")"=w300) -> ("States Out"=w299:string)  [unwired: 14 in]
      }
      frame "Macro: Initialize" {
        w302 = "Data: Initialize\nInitialize Core Data\nEvents: Register\nUI: Initialize\nUI: Front Panel State >> Open"  # Data: Initialize Initialize Core Data Events: Register UI: Initialize UI: Front Panel State >> Open
        # "#CSM \"Macro: Initialize\"\nInitialization Macro (This is called once, when the VI starts)"
        n90 = call <vilib>:"Add State(s) to Queue__JKI_lib_State_Machine.vi"("State(s) in Front (\"\")"=w302, "State(s) in (\"\")"=w306) -> ("States Out"=w305:string)  [unwired: 13 in]
      }
      frame "Macro: Exit" {
        # "#CSM \"Macro: Exit\"\nExit Macro (This is called once, when the VI exits)"
        n91 = Unbundle By Name(w314) -> ("Core.Close Panel on Exit?"=w313:bool)
        n92 = Select(t="UI: Front Panel State >> Close", s=w313, f="") -> (s? t:f=w310:string)
        n93 = call <vilib>:"Add State(s) to Queue__JKI_lib_State_Machine.vi"("State(s) in (\"\")"=w310, "State(s) at Back (\"\")"="Data: Cleanup\nEvents: Unregister\nExit") -> ("States Out"=w308:string)  [unwired: 13 in]
        n94 = call <vilib>:"Add State(s) to Queue__JKI_lib_State_Machine.vi"("State(s) in Front (\"\")"=w308, "State(s) in (\"\")"=w317) -> ("States Out"=w316:string)  [unwired: 13 in]
      }
      frame "---------- API ----------" {
        # "#CSM \"Category Seperator\"\nDo not put any code in this frame."
      }
      frame "API: API1" {
        # "#CSM API Example\nCopy/Rename this case for your own API"
        # "#CSM Response\nConnect this to return the response of your API"
        # "#CSM >> Source CSM >>\nIf you need to tell who triggered this state , use this string. If it's this case itself, this string is \"\"."
        # "#CSM >> Arguments >>\nDeal with the parameter if any"
      }
      frame "API: API2" {
        # "#CSM API Example\nCopy/Rename this case for your own API"
        # "unpack Hex String  to Variant\nif complex parameter is needed."
        n95 = call "CSM - Convert HexStr to Data.vi"("HEX String"=w328) -> ()  [unwired: 7 in, 2 out]
        n96 = disable-structure shown="Disabled" {
          disable-tunnel: [w333 "API2 Response"] -> w327
          frame Disabled {
            # "pack variant to hexstr \nif complex response is needed."
            # "complex Response"
            n97 = call "CSM - Convert Data to HexStr.vi"() -> ("HEX String (0-9,A-F)"=w333:string)  [unwired: 9 in]
          }
          frame Enabled {
          }
        }
      }
      frame "---------- DoSth ----------" {
        # "#CSM \"Category Seperator\"\nDo not put any code in this frame."
        n98 = call <vilib>:"Add State(s) to Queue__JKI_lib_State_Machine.vi"("State(s) in (\"\")"=w339) -> ("States Out"=w338:string)  [unwired: 14 in]
      }
      frame "DoSth: DoA" {
        # "#CSM \"Internal State\"\nThis category is used for holding internal states"
        n99 = call <vilib>:"Add State(s) to Queue__JKI_lib_State_Machine.vi"("State(s) in (\"\")"=w345) -> ("States Out"=w344:string)  [unwired: 14 in]
      }
      frame "DoSth: DoB" {
        # "#CSM \"Internal State\"\nThis category is used for holding internal states"
        n100 = call <vilib>:"Add State(s) to Queue__JKI_lib_State_Machine.vi"("State(s) in (\"\")"=w351) -> ("States Out"=w350:string)  [unwired: 14 in]
      }
    }
  }
